vi "HeaderAction.vi"(0 "InstrClass":refnum<class "AttoAMC.lvclass"> caption="DNL_LabVIEW Object in", 11 "error in (no error)":errorcluster caption="entrée d'erreur (pas d'erreur)") -> (4 "InstrClassOut":refnum<class "AttoAMC.lvclass"> caption="DNL_LabVIEW Object out", 6 "DataNames":string[](array[string]), 8 "Instr Name":string, 10 "HeaderString":string, 13 "ArrDatNames":string[](array[string]), 14 "DisplayNames":string[](array[string]), 15 "error out":errorcluster caption="sortie d'erreur")   [LabVIEW 2019, in "AttoAMC.lvclass"]
uses:
  AttoAMC.lvclass
  C:/Programmes Labview/LabscanV1A/DevicesClass/BaseDevice/BaseDevice.lvclass
  AttoAMC.lvclass/AttoAMC.ctl
  <userlib>/GenProg/ReadValByRefBool.vi
  <vilib>/Utility/error.llb/Error Cluster From Error Code.vi
  <vilib>/ErrorRing/Error Ring.xnode
  BaseDevice/BaseDevice.lvclass
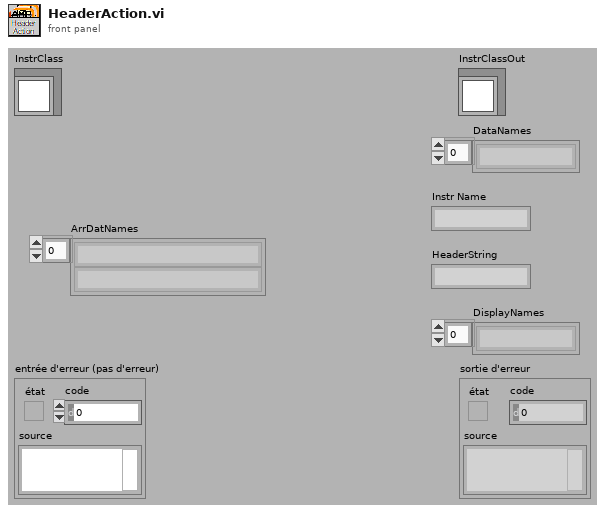
[diagram p1: front panel]
types:
  T1 = typedef "AttoAMC.lvclass/AttoAMC_Func.ctl" = enum16{"Position (um)"}
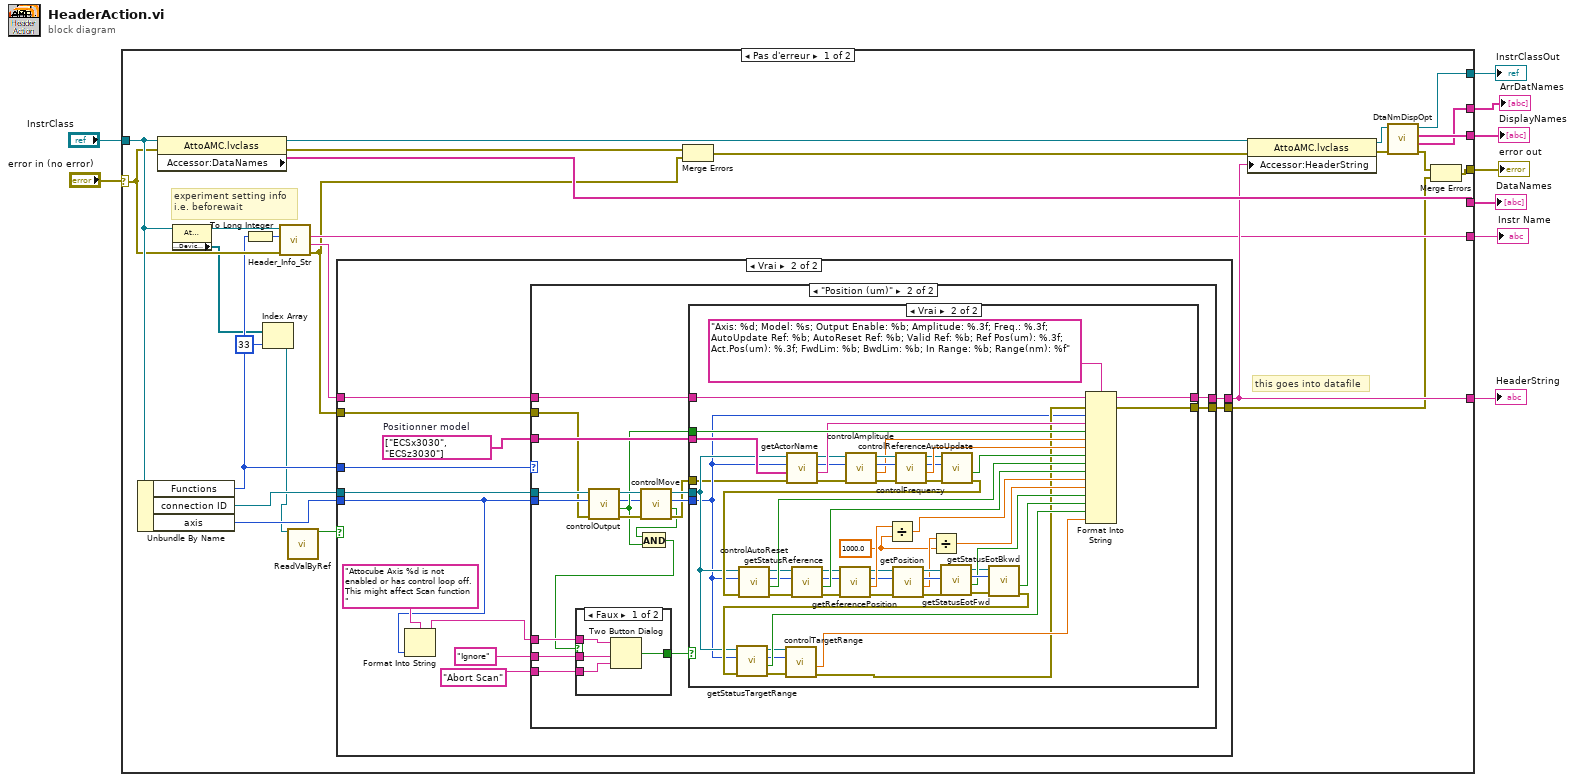
[diagram p0: block diagram]
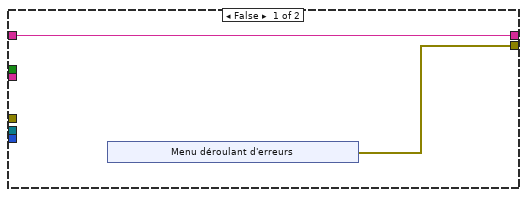
[diagram p5: hidden frame]
diagram:
  n1 = case shown="Pas d'erreur" "error in (no error)" {
    selector: "error in (no error)" -> [w26 w139]
    tunnel: [w33 _] -> w8
    tunnel: [w36 _] -> w7
    tunnel: "InstrClass" -> [w29 w140]
    tunnel: [w22 w139] -> w5
    tunnel: [w20 w140] -> w3
    tunnel: [w28 _] -> w4
    tunnel: [w30 _] -> w2
    tunnel: [w18 _] -> w1
    frame No Error {
      # "this goes into datafile"
      # "experiment setting info\ni.e. beforewait"
      n2 = Unbundle By Name(w29) -> ("Functions"=w24:T1, "connection ID"=w17:refnum<k5>, "axis"=w16:u8)
      n3 = property class="AttoAMC.lvclass"(reference=w29, error in=w26) -> (reference out=w35:refnum<class "AttoAMC.lvclass">, error out=w34:errorcluster, "Accessor:DataNames"=w36:string[])
      n4 = property class="AttoAMC.lvclass"(reference=w29) -> (reference out=w14:refnum<class "AttoAMC.lvclass">, "Accessor:DeviceCtrl"=w13:refnum<vi>[])  [unwired: 1 in, 1 out]
      n5 = To Long Integer(number=w24) -> (32bit integer=w23:i32)
      n6 = Index Array(array=w13, index=33 ("indice")) -> (element=w11:refnum<vi>)
      n7 = call-dynamic "Header_Info_Str.vi"("error in (no error)"=w26, "Functions"=w23, "DefaultDev in"=w14) -> ("error out"=w15:errorcluster, "HdrInfoStr"=w27:string, "InstrumentName"=w28:string)  [unwired: 5 in, 1 out]
      n8 = call-poly <userlib>:"ReadValByRef.vi"("Control Ref"=w11) -> ("Valeur"=w10:bool)  [unwired: 13 in, 1 out]
      n9 = case shown="Vrai" w10 {
        tunnel: [w38 w50] -> w33
        tunnel: w27 -> [w38 w49]
        tunnel: w24 -> [_ w48]
        tunnel: [w37 w47] -> w21
        tunnel: w17 -> [_ w46]
        tunnel: w16 -> [_ w43]
        tunnel: w15 -> [w37 w45]
        frame False {
        }
        frame True {
          w39 = string[] ["ECSx3030", "ECSz3030"]  # Positionner model
          n10 = Format Into String(format string="Attocube Axis %d is not enabled or has control loop off. This might affect Scan function " ("message"), w43) -> (resulting string=w40:string)  [unwired: 2 in, 1 out]
          n11 = case shown="\"Position (um)\"" w48 {
            tunnel: [w52 w70] -> w50
            tunnel: w49 -> [w52 w71]
            tunnel: w39 -> [_ w72]
            tunnel: w43 -> [_ w64]
            tunnel: w46 -> [_ w67]
            tunnel: w45 -> [w51 w63]
            tunnel: [w51 w69] -> w47
            tunnel: w40 -> [_ w57]
            tunnel: "Abort Scan" ("Nom du bouton F (\"Annuler\")") -> [_ w56]
            tunnel: "Ignore" ("Nom du bouton V (\"OK\")") -> [_ w55]
            frame Default {
            }
            frame "Position (um)" {
              n12 = call <userlib>:"controlOutput.vi"("error in"=w63, "axis in"=w64, "connection ID"=w67) -> ("error out"=w62:errorcluster, "enable output out"=w59:bool, "axis out"=w53:u8, "connection ID"=w68:refnum<k5>)  [unwired: 5 in]
              n13 = call <userlib>:"controlMove.vi"("error in"=w62, "axis in"=w53, "connection ID"=w68) -> ("error out"=w61:errorcluster, "controll move out"=w60:bool, "axis out"=w65:u8, "connection ID"=w66:refnum<k5>)  [unwired: 5 in]
              n14 = And(x=w60, y=w59) -> (x .and. y?=w54:bool)
              n15 = case shown="Faux" w54 {
                selector: w54 -> [_ w77]
                tunnel: [w76 w77] -> w58
                tunnel: w57 -> [w75 _]
                tunnel: w56 -> [w74 _]
                tunnel: w55 -> [w73 _]
                frame False {
                  n16 = Two Button Dialog(message=w75, 1:w74, 2:w73) -> (T button?=w76:bool)
                }
                frame True {
                }
              }
              n17 = case shown="Vrai" w58 {
                tunnel: w72 -> [_ w138]
                tunnel: w71 -> [w79 w137]
                tunnel: w59 -> [_ w135]
                tunnel: [w79 w100] -> w70
                tunnel: [w78 w94] -> w69
                tunnel: w66 -> [_ w87]
                tunnel: w65 -> [_ w86]
                tunnel: w61 -> [_ w85]
                frame False {
                  n18 = xnode "Menu déroulant d'erreurs"() -> ("sortie d'erreur"=w78:errorcluster)
                }
                frame True {
                  w96 = 1000.0 ("y")
                  n19 = call <userlib>:"getActorName.vi"("error in"=w85, "Actor Names"=w138, "axis in"=w86, "connection ID"=w87) -> ("error out"=w90:errorcluster, "ActorName out"=w92:string, "axis out"=w88:u8, "connection ID"=w89:refnum<k5>)  [unwired: 4 in]
                  n20 = call <userlib>:"controlAmplitude.vi"("error in"=w90, "axis in"=w88, "connection ID"=w89) -> ("error out"=w132:errorcluster, "amplitude [V] out"=w131:dbl, "axis out"=w134:u8, "connection ID"=w133:refnum<k5>)  [unwired: 5 in]
                  n21 = call <userlib>:"controlFrequenzy.vi"("error in"=w132, "axis in"=w134, "connection ID"=w133) -> ("error out"=w129:errorcluster, "Frequenzy [Hz] out"=w130:dbl, "axis out"=w127:u8, "connection ID"=w128:refnum<k5>)  [unwired: 5 in]
                  n22 = call <userlib>:"controlReferenceAutoUpdate.vi"("error in"=w129, "axis in"=w127, "connection ID"=w128) -> ("error out"=w125:errorcluster, "ref auto up out"=w126:bool)  [unwired: 5 in, 2 out]
                  n23 = call <userlib>:"controlAutoReset.vi"("error in"=w125, "axis in"=w86, "connection ID"=w87) -> ("error out"=w121:errorcluster, "auto reset out"=w124:bool, "axis out"=w122:u8, "connection ID"=w123:refnum<k5>)  [unwired: 5 in]
                  n24 = call <userlib>:"getStatusReference.vi"("error in"=w121, "axis in"=w122, "connection ID"=w123) -> ("error out"=w117:errorcluster, "status reference out"=w120:bool, "axis out"=w115:u8, "connection ID"=w116:refnum<k5>)  [unwired: 5 in]
                  n25 = call <userlib>:"getReferencePosition.vi"("error in"=w117, "axis in"=w115, "connection ID"=w116) -> ("error out"=w107:errorcluster, "Reference position out"=w119:dbl, "axis out"=w105:u8, "connection ID"=w106:refnum<k5>)  [unwired: 5 in]
                  n26 = Divide(x=w119, y=w96) -> (x/y=w118:dbl)
                  n27 = call <userlib>:"getPosition.vi"("error in"=w107, "axis in"=w105, "connection ID"=w106) -> ("error out"=w113:errorcluster, "position out"=w108:dbl, "axis out"=w112:u8, "connection ID"=w114:refnum<k5>)  [unwired: 5 in]
                  n28 = Divide(x=w108, y=w96) -> (x/y=w104:dbl)
                  n29 = call <userlib>:"getStatusEotFwd.vi"("error in"=w113, "axis in"=w112, "connection ID"=w114) -> ("error out"=w111:errorcluster, "Status EOT FWD out"=w103:bool, "axis out"=w109:u8, "connection ID"=w93:refnum<k5>)  [unwired: 5 in]
                  n30 = call <userlib>:"getStatusEotBkwd.vi"("error in"=w111, "axis in"=w109, "connection ID"=w93) -> ("error out"=w110:errorcluster, "Get Stus EOT BKWD out"=w102:bool)  [unwired: 5 in, 2 out]
                  n31 = call <userlib>:"getStatusTargetRange.vi"("error in"=w110, "axis in"=w86, "connection ID"=w87) -> ("error out"=w98:errorcluster, "Status Target Range out"=w101:bool, "axis out"=w97:u8, "connection ID"=w99:refnum<k5>)  [unwired: 5 in]
                  n32 = call <userlib>:"controlTargetRange.vi"("error in"=w98, "axis in"=w97, "connection ID"=w99) -> ("error out"=w91:errorcluster, "Target Range out"=w95:dbl)  [unwired: 5 in, 2 out]
                  n33 = Format Into String(format string="Axis: %d; Model: %s; Output Enable: %b; Amplitude: %.3f; Freq.: %.3f; AutoUpdate Ref: %b; AutoReset Ref: %b; Valid Ref: %b; Ref Pos(um): %.3f; Act.Pos(um): %.3f; FwdLim: %b; BwdLim: %b; In Range: %b; Range(nm): %f" ("chaîne de format"), initial string=w137, error in=w91, w86, w92, w135, w131, w130, w126, w124, w120, w118, w104, w103, w102, w101, w95) -> (resulting string=w100:string, error out=w94:errorcluster)
                }
              }
            }
          }
        }
      }
      n34 = Merge Errors(w34, w15) -> (w25:errorcluster)
      n35 = property class="AttoAMC.lvclass"(reference=w35, error in=w25, "Accessor:HeaderString"=w33) -> (reference out=w31:refnum<class "AttoAMC.lvclass">, error out=w32:errorcluster)
      n36 = call "DtaNmDispOpt.vi"("error in (no error)"=w32, "BaseDevice en entrée"=w31) -> ("error out"=w19:errorcluster, "ArrDisplayNames"=w18:string[], "DisplayNames"=w30:string[], "BaseDevice en sortie"=w20:refnum<class "AttoAMC.lvclass">)  [unwired: 6 in]
      n37 = Merge Errors(w19, w21) -> (w22:errorcluster)
    }
    frame Error {
    }
  }
  "error out" <- w5
  "InstrClassOut" <- w3
  "DataNames" <- w7
  "HeaderString" <- w8
  "Instr Name" <- w4
  "DisplayNames" <- w2
  "ArrDatNames" <- w1
